vi "numerical-integration-test.vi"(8 "error in (no error)":errorcluster) -> (0 "error out":errorcluster, 3 "All passed":bool)   [LabVIEW 2019]
uses:
  <vilib>/Analysis/Matrix/Datatypes/RealMatrix.ctl
  <vilib>/Rock Robotics/WPI/ThirdParty/JAS_Junk/TrajLib/MatBuilder_Create.vi
  <vilib>/Rock Robotics/WPI/ThirdParty/JAS_Junk/TrajLib/Trajectory_Library.lvlib
  <vilib>/Analysis/Matrix/NI_Matrix.lvlib
panel:
  out "Output Test 2":dbl
  out "Output Test 1":dbl
  out "Passed 2":bool
  out "Error 2":bool
  out "Test 2":T1
  out "Passed 1":bool
  out "Error 1":bool
  out "Test 1":T1
  out "Passed  0":bool
  out "Error 0":bool
  out "Test 0":T1
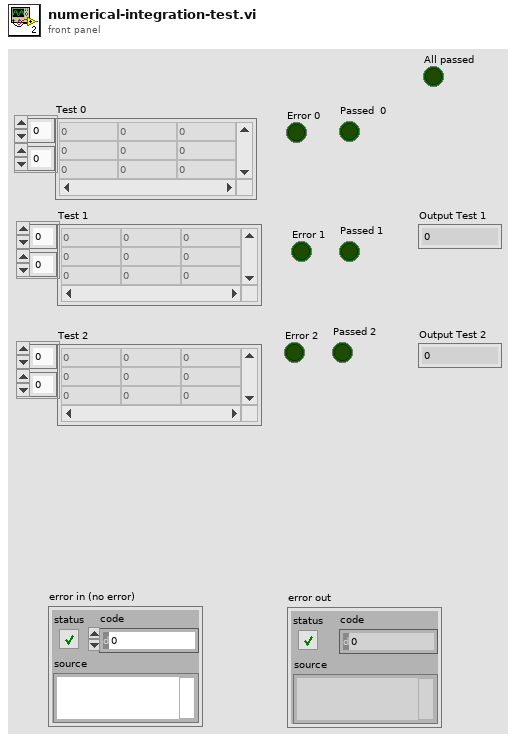
[diagram p1: front panel]
types:
  T1 = typedef "NI_Matrix.lvlib/RealMatrix.ctl" = dbl[][]
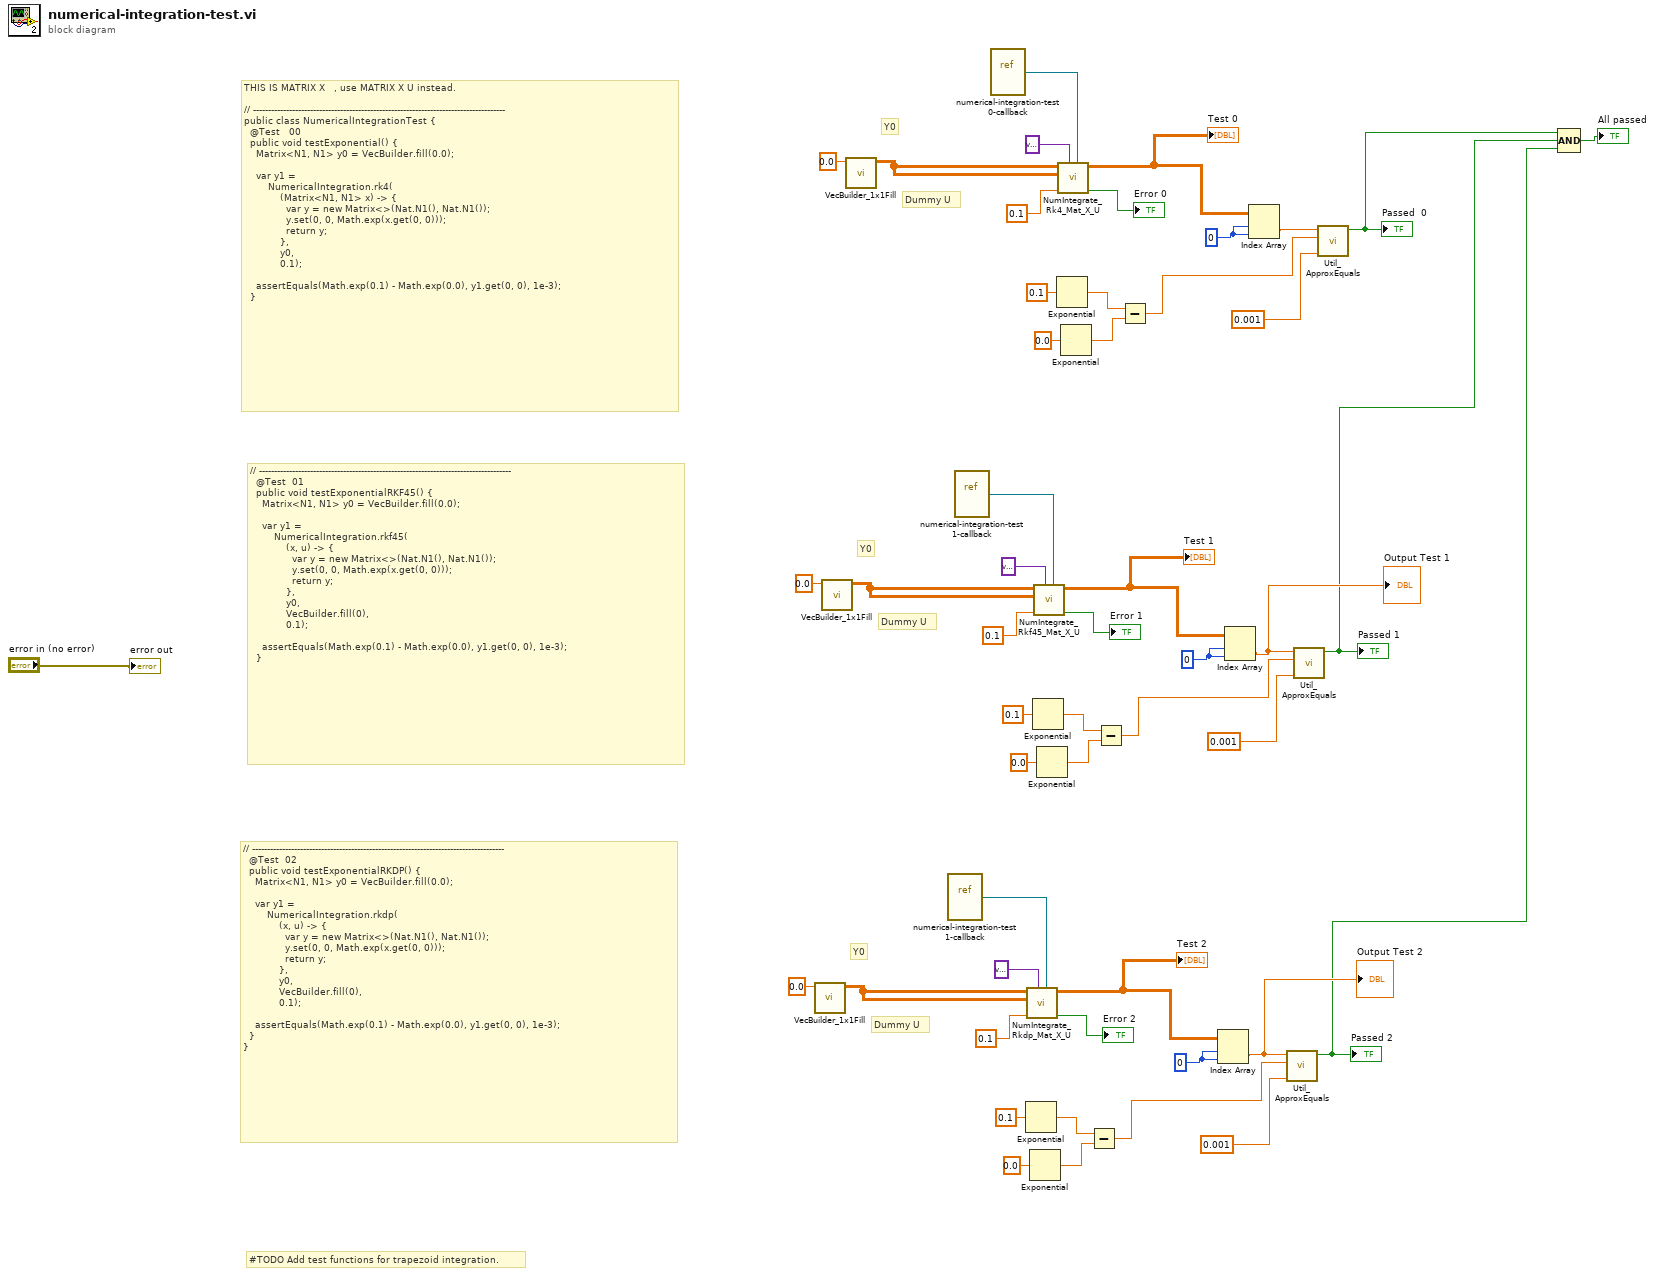
[diagram p0: block diagram]
diagram:
  w11 = 0 ("index (row)")
  w30 = 0 ("index (row)")
  w44 = 0 ("index (row)")
  # "Dummy U"
  # "Y0"
  # "#TODO Add test functions for trapezoid integration."
  # "Dummy U"
  # "Y0"
  # "Dummy U"
  # "Y0"
  # "// ------------------------------------------------------------------------------------\n  @Test  01\n  public void testExponentialRKF45() {\n    Matrix<N1, N1> y0 = VecBuilder.fill(0.0);\n\n    var y1 =\n        NumericalIntegration.rkf45(\n            (x, u) -> {\n              var y = new Matrix<>(Nat.N1(), Nat.N1());\n              y.set(0, 0, Math.exp(x.get(0, 0)));\n              return y;\n            },\n            y0,\n            VecBuilder.fill(0),\n            0.1);\n\n    assertEquals(Math.exp(0.1) - Math.exp(0.0), y1.get(0, 0), 1e-3);\n  }"
  # "THIS IS MATRIX X   , use MATRIX X U instead.\n\n// ------------------------------------------------------------------------------------\npublic class NumericalIntegrationTest {\n  @Test   00\n  public void testExponential() {\n    Matrix<N1, N1> y0 = VecBuilder.fill(0.0);\n\n    var y1 =\n        NumericalIntegration.rk4(\n            (Matrix<N1, N1> x) -> {\n              var y = new Matrix<>(Nat.N1(), Nat.N1());\n              y.set(0, 0, Math.exp(x.get(0, 0)));\n              return y;\n            },\n            y0,\n            0.1);\n\n    assertEquals(Math.exp(0.1) - Math.exp(0.0), y1.get(0, 0), 1e-3);\n  }"
  # "// ------------------------------------------------------------------------------------\n  @Test  02\n  public void testExponentialRKDP() {\n    Matrix<N1, N1> y0 = VecBuilder.fill(0.0);\n\n    var y1 =\n        NumericalIntegration.rkdp(\n            (x, u) -> {\n              var y = new Matrix<>(Nat.N1(), Nat.N1());\n              y.set(0, 0, Math.exp(x.get(0, 0)));\n              return y;\n            },\n            y0,\n            VecBuilder.fill(0),\n            0.1);\n\n    assertEquals(Math.exp(0.1) - Math.exp(0.0), y1.get(0, 0), 1e-3);\n  }\n}"
  n1 = call <vilib>:"VecBuilder_1x1Fill.vi"("R0_C0"=0.0) -> ("output matrix"=w14:T1)  [unwired: 10 in]
  n2 = call <vilib>:"VecBuilder_1x1Fill.vi"("R0_C0"=0.0) -> ("output matrix"=w33:T1)  [unwired: 10 in]
  n3 = call <vilib>:"VecBuilder_1x1Fill.vi"("R0_C0"=0.0) -> ("output matrix"=w48:T1)  [unwired: 10 in]
  n4 = vi-ref "numerical-integration-test1-callback.vi"() -> (w3:refnum<vi>)
  n5 = vi-ref "numerical-integration-test1-callback.vi"() -> (w18:refnum<vi>)
  n6 = vi-ref "numerical-integration-test0-callback.vi"() -> (w45:refnum<vi>)
  n7 = Exponential(1:0.1 ("x")) -> (0:w5:dbl)
  n8 = call <vilib>:"NumIntegrate_Rkdp_Mat_X_U.vi"("Func_X_U_Extra"=w3, "PassedData"=variant, "dT_Seconds"=0.1, "U"=w14, "X"=w14) -> ("Error"=→"Error 2":bool, "Return X"=w10:T1)  [unwired: 4 in, 1 out]
  "Test 2" <- w10
  n9 = Exponential(1:0.0 ("x")) -> (0:w4:dbl)
  n10 = Exponential(1:0.1 ("x")) -> (0:w23:dbl)
  n11 = call <vilib>:"NumIntegrate_Rkf45_Mat_X_U.vi"("Func_X_U_Extra"=w18, "PassedData"=variant, "dT_Seconds"=0.1, "U"=w33, "X"=w33) -> ("Error"=→"Error 1":bool, "Return X"=w29:T1)  [unwired: 4 in, 1 out]
  "Test 1" <- w29
  n12 = Exponential(1:0.0 ("x")) -> (0:w22:dbl)
  n13 = Exponential(1:0.1 ("x")) -> (0:w37:dbl)
  n14 = call <vilib>:"NumIntegrate_Rk4_Mat_X_U.vi"("Func_X_U_Extra"=w45, "PassedData"=variant, "dT_Seconds"=0.1, "U"=w48, "X"=w48) -> ("Error"=→"Error 0":bool, "OUTPUT"=w43:T1)  [unwired: 5 in]
  "Test 0" <- w43
  n15 = Exponential(1:0.0 ("x")) -> (0:w36:dbl)
  n16 = Subtract(x=w5, y=w4) -> (x-y=w6:dbl)
  n17 = Subtract(x=w23, y=w22) -> (x-y=w24:dbl)
  n18 = Subtract(x=w37, y=w36) -> (x-y=w38:dbl)
  n19 = Index Array(array=w10, index (row)=w11, index (col)=w11) -> (element=w2:dbl)
  "Output Test 2" <- w2
  n20 = Index Array(array=w29, index (row)=w30, index (col)=w30) -> (element=w27:dbl)
  "Output Test 1" <- w27
  n21 = Index Array(array=w43, index (row)=w44, index (col)=w44) -> (element=w41:dbl)
  n22 = call <vilib>:"Util_ApproxEquals.vi"("Tolerance"=0.001, "Value 2"=w6, "Value 1"=w2) -> ("ApproxEquals"=w1:bool)  [unwired: 8 in]
  "Passed 2" <- w1
  n23 = call <vilib>:"Util_ApproxEquals.vi"("Tolerance"=0.001, "Value 2"=w24, "Value 1"=w27) -> ("ApproxEquals"=w20:bool)  [unwired: 8 in]
  "Passed 1" <- w20
  n24 = call <vilib>:"Util_ApproxEquals.vi"("Tolerance"=0.001, "Value 2"=w38, "Value 1"=w41) -> ("ApproxEquals"=w21:bool)  [unwired: 8 in]
  "Passed  0" <- w21
  n25 = Compound Arithmetic op=AND(w21, w20, w1) -> (→"All passed":bool)
  "error out" <- "error in (no error)"
